vi "Internal Transition.vi"(8 "error in (no error)":errorcluster, 11 "_State Machine Actor in":refnum<class "_State Machine Actor.lvclass">) -> (0 "error out":errorcluster, 3 "_State Machine Actor out":refnum<class "_State Machine Actor.lvclass">)   [LabVIEW 2024, in "_State Machine Actor.lvlib" / "_State Machine Actor.lvclass"]
uses:
  _State Machine Actor.lvclass
  _State Machine Actor.lvclass/_State Machine Actor.ctl
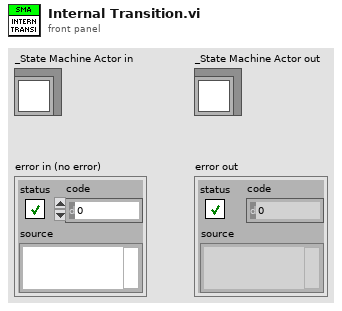
[diagram p1: front panel]
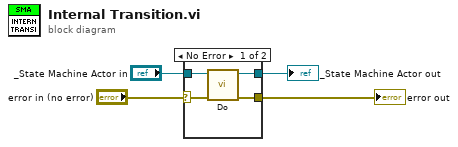
[diagram p0: block diagram]
diagram:
  n1 = case shown="No Error" "error in (no error)" {
    selector: "error in (no error)" -> [w6 w10]
    tunnel: [w5 w10] -> w3
    tunnel: [w7 w9] -> w1
    tunnel: "_State Machine Actor in" -> [w8 w9]
    frame No Error {
      n2 = call-dynamic "Do.vi"("error in (no error)"=w6, "_State Machine Actor in"=w8) -> ("error out"=w5:errorcluster, "_State Machine Actor out"=w7:refnum<class "_State Machine Actor.lvclass">)  [unwired: 8 in]
    }
    frame Error {
    }
  }
  "error out" <- w3
  "_State Machine Actor out" <- w1
